vi "Editor UI.vi"(8 "error in (no error)":errorcluster, 11 "Recipe Editor in":refnum<class "Recipe Editor.lvclass">) -> (0 "error out":errorcluster, 3 "Recipe Editor out":refnum<class "Recipe Editor.lvclass">)   [LabVIEW 2018, in "Temp Recipe.lvlib" / "Recipe Editor.lvclass"]
uses:
  Recipe Editor.lvclass
  Recipe Editor.lvclass/Recipe Editor.ctl
  Update Event Data.ctl
  Libraries/OOPanel/OOPanel/PanelArray/PanelArray.lvclass
  Libraries/OOPanel/OOPanel/Panel/Panel.lvclass
  Temp Recipe.lvlib
panel:
  in  "Ambient":dbl format="%.1f °F"
  in  "New Step":bool
  out "Preview":cluster{"Time":dbl[], "Value":dbl[]}(graph)
  in  "Scrollbar":i32(c297)
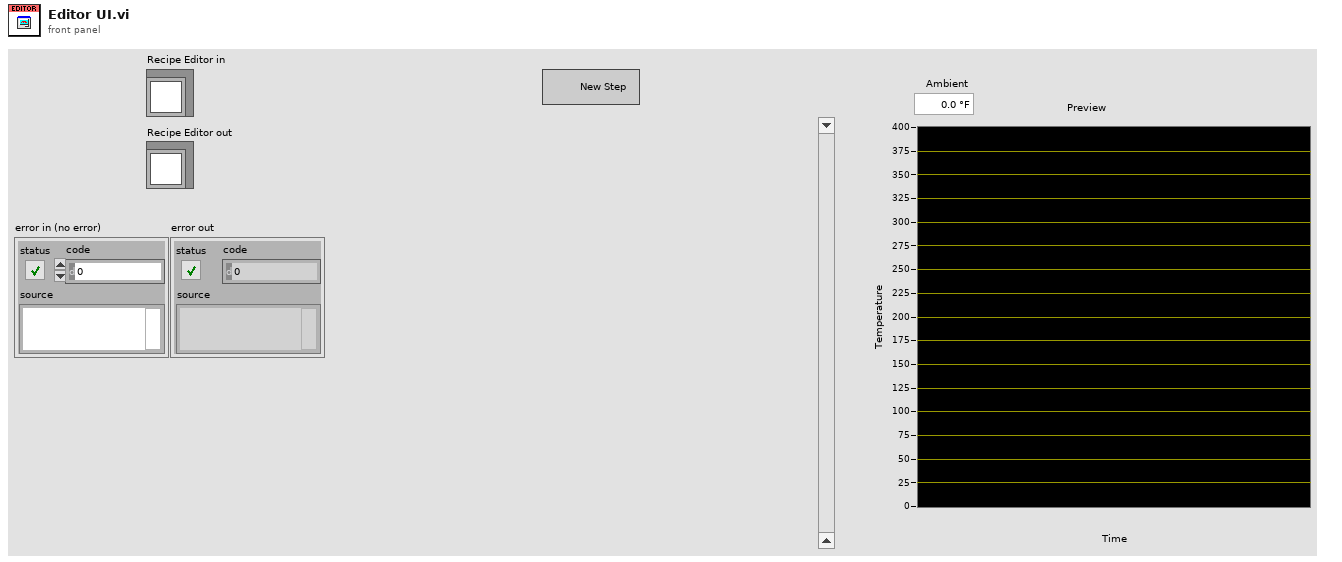
[diagram p1: front panel]
types:
  T1 = typedef "Temp Recipe.lvlib/Update Event Data.ctl" = bool
  T2 = typedef "Temp Recipe.lvlib/Recipe Editor.lvclass/Step Type.ctl" = enum16{"Setpoint", "Step Rate", "Rate Duration", "Delay"}
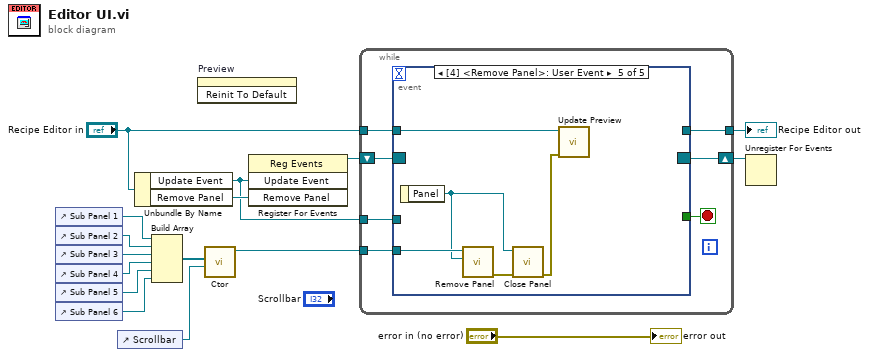
[diagram p0: block diagram]
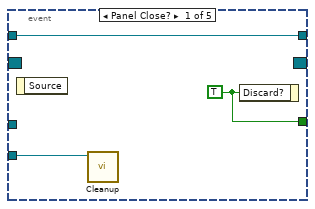
[diagram p2: hidden frame]
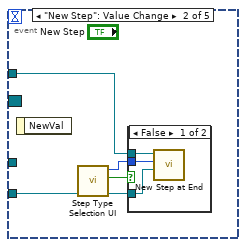
[diagram p3: hidden frame]
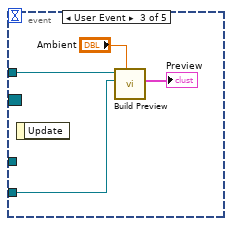
[diagram p5: hidden frame]
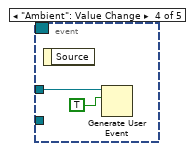
[diagram p6: hidden frame]
diagram:
  n1 = control-ref of="Sub Panel 1"() -> (w14:refnum<vi>)
  n2 = control-ref of="Sub Panel 2"() -> (w15:refnum<vi>)
  n3 = control-ref of="Sub Panel 3"() -> (w16:refnum<vi>)
  n4 = control-ref of="Sub Panel 4"() -> (w13:refnum<vi>)
  n5 = control-ref of="Sub Panel 5"() -> (w12:refnum<vi>)
  n6 = control-ref of="Sub Panel 6"() -> (w11:refnum<vi>)
  n7 = control-ref of="Scrollbar"() -> (w9:refnum<vi>)
  n8 = Unbundle By Name("Recipe Editor in") -> ("Update Event"=w1:refnum<user-event>, "Remove Panel"=w2:refnum<user-event>)
  n9 = Build Array(w14, w15, w16, w13, w12, w11) -> (w10:refnum<vi>[])
  n10 = invoke on="Preview" class="XYGraph (strict)" method="Reinit To Default"() -> ()  [unwired: 3 in, 3 out]
  n11 = call "Ctor.vi"("Scrollbar"=w9, "SubPanels"=w10) -> ("PanelArray out"=w8:refnum<class "PanelArray.lvclass">)  [unwired: 8 in, 1 out]
  n12 = register-events(w1, w2) -> (reference out=w6:refnum<event-registration>)  [unwired: 2 in, 1 out]
  n13 = while {
    tunnel: w8 -> [w23]
    tunnel: "Recipe Editor in" -> [w22]
    shift-right: [w19] -> w5
    shift-left: w6 -> [w20]
    tunnel: [w18] -> w4
    tunnel: w1 -> [w17]
    stop <- w21 stop-if-true
    n14 = event shown="[4] <Remove Panel>: User Event" {
      selector: w20 -> [_ _ _ _ _]
      dyn-events: [_ _ _ _ _] -> w19
      timeout: _ -> [_ _ _ _ _]
      tunnel: w23 -> [w25 w27 w35 _ w44]
      tunnel: w22 -> [w24 w29 w37 _ w40]
      tunnel: [w26 _ _ _ _] -> w21
      tunnel: [w24 _ _ _ _] -> w18
      tunnel: w17 -> [_ _ _ w39 _]
      event Panel Close? {
        w26 = TRUE ("Discard?")
        n15 = event-data() -> ()  [unwired: 1 in, 1 out]
        n16 = call "Cleanup.vi"("PanelArray in"=w25) -> ()  [unwired: 10 in, 1 out]
        n17 = event-data("Discard?"=w26) -> ()  [unwired: 1 in, 1 out]
      }
      event "New Step": Value Change {
        n18 = event-data() -> ()  [unwired: 1 in, 1 out]
        n19 = call "Step Type Selection UI.vi"() -> ("Cancelled"=w30:bool, "Step Type"=w28:T2)  [unwired: 10 in]
        n20 = case shown="False" w30 {
          tunnel: w29 -> [w33 _]
          tunnel: w28 -> [w32 _]
          tunnel: w27 -> [w31 _]
          frame False {
            n21 = call "New Step at End.vi"("PanelArray"=w31, "Step Type"=w32, "Recipe Editor in"=w33) -> ()  [unwired: 7 in, 2 out]
          }
          frame True {
          }
        }
      }
      event User Event {
        n22 = event-data() -> ()  [unwired: 1 in, 1 out]
        n23 = call "Build Preview.vi"("Ambient"="Ambient", "PanelArray"=w35, "Recipe Editor in"=w37) -> ("Step Plot Data"=→"Preview":cluster{"Time":dbl[], "Value":dbl[]})  [unwired: 6 in, 2 out]
      }
      event "Ambient": Value Change {
        n24 = event-data() -> ()  [unwired: 1 in, 1 out]
        n25 = Generate User Event(user event=w39, event data cluster=T1 TRUE ("event data")) -> ()  [unwired: 2 in, 2 out]
      }
      event User Event {
        n26 = event-data() -> ("Panel"=w42:refnum<class "Panel.lvclass">)  [unwired: 1 in]
        n27 = call "Remove Panel.vi"("Panel"=w42, "PanelArray in"=w44) -> ("error out"=w43:errorcluster)  [unwired: 8 in, 1 out]
        n28 = call "Close Panel.vi"("error in (no error)"=w43, "Panel in"=w42) -> ("error out"=w41:errorcluster)  [unwired: 8 in, 1 out]
        n29 = call "Update Preview.vi"("error in (no error)"=w41, "Recipe Editor in"=w40) -> ()  [unwired: 8 in, 2 out]
      }
    }
  }
  "Recipe Editor out" <- w4
  n30 = Unregister For Events(event registration refnum=w5) -> ()  [unwired: 1 in, 1 out]
  "error out" <- "error in (no error)"
